vi "PID w reset.vi"(4 "State":i16, 5 "Time":dbl format="%.2f", 6 "Sensor Values":dbl[](array[numeric]), 7 "Set Points":dbl[](array[numeric])) -> (0 "required data":T1={"Set Point names"=["target value", "P Kc", "I Ti (min)", "D Td (min)"], "required number of setpoints"=4, "required number of sensors"=1, "Sensor names"=["Measured process value"]}, 3 "output value":dbl)   [LabVIEW 2012]
uses:
  PID library.llb/PID (DBL).vi
panel:
  # "Enter the correct information for this control code in the required data structure below. Then make the current value default by right clicking on the border of the data structure."
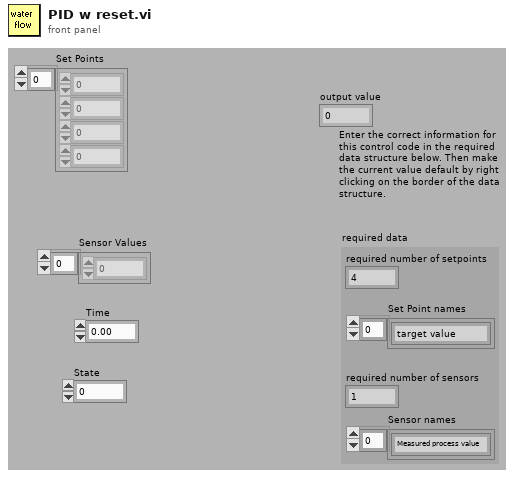
[diagram p1: front panel]
types:
  T1 = cluster{"Set Point names":string[], "required number of setpoints":u8, "required number of sensors":u8, "Sensor names":string[]}
  T2 = cluster{"Set Points[0]":dbl, "Set Points[1]":dbl, "Set Points[2]":dbl, "Set Points[3]":dbl}
  T3 = cluster{"Set Points[1]":dbl, "Set Points[2]":dbl, "Set Points[3]":dbl}
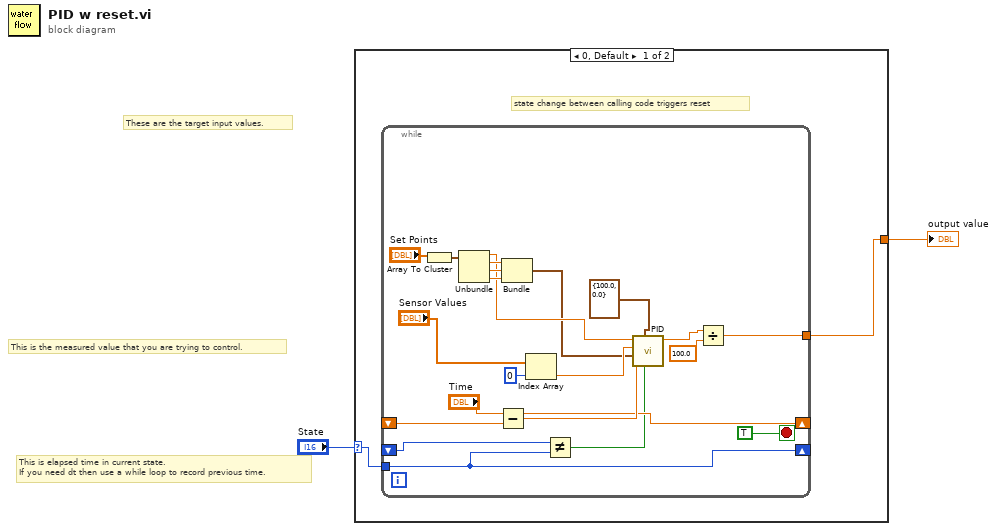
[diagram p0: block diagram]
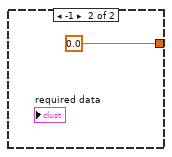
[diagram p2: hidden frame]
diagram:
  # "These are the target input values."
  # "This is the measured value that you are trying to control."
  # "This is elapsed time in current state.\nIf you need dt then use a while loop to record previous time."
  n1 = case shown="0, Default" "State" {
    selector: "State" -> [w3 _]
    tunnel: [w4 0.0 ("fraction on")] -> w2
    frame 0, Default {
      # "state change between calling code triggers reset"
      n2 = while {
        shift-right: ["Time"] -> _
        shift-left: _ -> [w24]
        tunnel: [w18] -> w4
        shift-right: [w8] -> _
        shift-left: _ -> [w9]
        tunnel: w3 -> [w8]
        stop <- TRUE stop-if-true
        n3 = Array To Cluster(array="Set Points") -> (cluster=w17:T2)
        n4 = Unbundle(w17) -> ("Set Points[0]"=w10:dbl, "Set Points[1]"=w15:dbl, "Set Points[2]"=w16:dbl, "Set Points[3]"=w14:dbl)
        n5 = Subtract(x="Time", y=w24) -> (x-y=w23:dbl)
        n6 = Bundle("Set Points[1]"=w15, "Set Points[2]"=w16, "Set Points[3]"=w14) -> (w6:T3)  [unwired: 1 in]
        n7 = Index Array(array="Sensor Values", index=0) -> (element=w11:dbl)
        n8 = Not Equal?(x=w9, y=w8) -> (x != y?=w7:bool)
        n9 = call-poly "PID.vi"("reinitialize? (F)"=w7, "output range"=cluster{"output high":dbl, "output low":dbl} {"output high"=100.0, "output low"=0.0}, "dt (s)"=w23, "PID gains"=w6, "process variable"=w11, "setpoint"=w10) -> ("output"=w21:dbl)  [unwired: 4 in, 1 out]
        n10 = Divide(x=w21, y=100.0) -> (x/y=w18:dbl)
      }
    }
    frame -1 {
    }
  }
  "output value" <- w2
